vi "TEiSO2-43i_new_config_file.vi"() -> ()   [LabVIEW 2014]
panel:
  out "error out":errorcluster
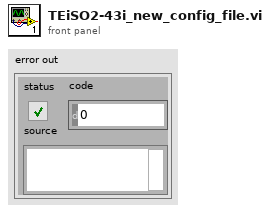
[diagram p1: front panel]
types:
  T1 = enum16{"open", "replace", "create", "open or create", "replace or create", "replace or create with confirmation"}
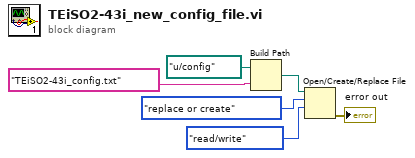
[diagram p0: block diagram]
diagram:
  n1 = Build Path(base path=path "u:/config", name or relative path="TEiSO2-43i_config.txt" ("string")) -> (appended path=w3:path)
  n2 = Open/Create/Replace File(file path (use dialog)=w3, operation (0:open)=T1."replace or create", access (0:read/write)=enum16{"read/write", "read-only", "write-only"}."read/write") -> (error out=→"error out":errorcluster)  [unwired: 3 in, 2 out]
